vi "cRIO_FPGA_COMMUNICATION  Schreibe Werte für eine Station.vi"(8 "Fehler (Eingang, kein Fehler)":errorcluster, 9 "Stationen":bool[][](array[boolean]), 10 "Bänder":bool[][](array[boolean]), 11 "FPGA-VI-Referenz (Ausgang)":refnum<k20>) -> (0 "Fehler (Ausgang)":errorcluster)   [LabVIEW 2013, in "cRIO_FPGA_COMMUNICATION.lvlib"]
uses:
  cRIO_FPGA_COMMUNICATION.lvlib
  <vilib>/Utility/error.llb/Error Cluster From Error Code.vi
  <vilib>/rvi/errors/niLvFpgaAdjustHostInterfaceError.vi
  <vilib>/rvi/interface/nirviReadWriteControl/nirviReadWriteControl.xnode
  FPGA Bitfiles/Test_FPGATarget_CScRIOPBFPGADP-M_4E0AD52E.lvbitx
  NiFpgaLv.dll
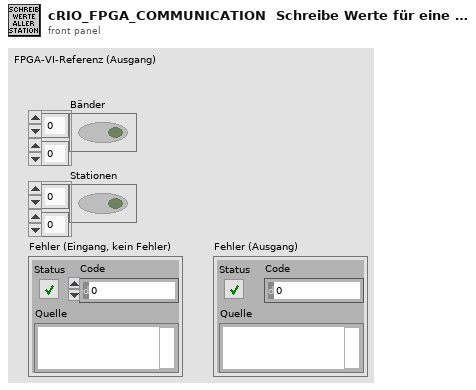
[diagram p1: front panel]
types:
  T1 = enum16{"Init", "Zählerkonfig. setzen", "lese Zählerkonfig."}
  T2 = enum16{"Init", "Zählerwert nullen", "Zählerwert setzen", "lese gesetzten Zählerwert"}
  T3 = cluster{"Index (Station/Band)":u8, "Station/Band":enum16{"Station", "Band"}, "Bitstelle":u8, "Zählrichtung":enum16{"Hochzählen", "Runterzählen"}}[]
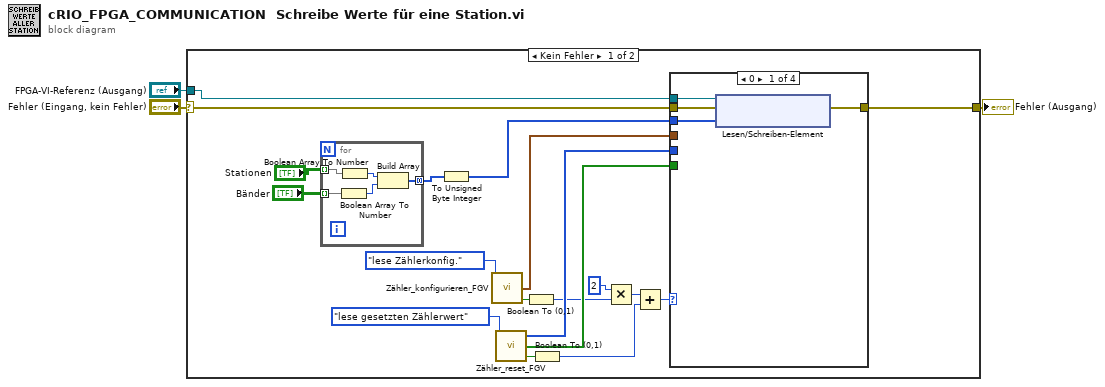
[diagram p0: block diagram]
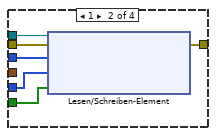
[diagram p2: hidden frame]
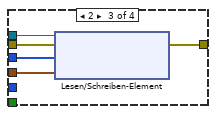
[diagram p3: hidden frame]
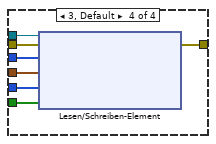
[diagram p4: hidden frame]
diagram:
  n1 = case shown="Kein Fehler" "Fehler (Eingang, kein Fehler)" {
    selector: "Fehler (Eingang, kein Fehler)" -> [w17 w50]
    tunnel: [w18 w50] -> w3
    tunnel: "FPGA-VI-Referenz (Ausgang)" -> [w16 _]
    frame No Error {
      n2 = for {
        tunnel: "Bänder" -> [w49] mode=indexing
        tunnel: "Stationen" -> [w48] mode=indexing
        tunnel: [w45] -> w20 mode=concatenating
        n3 = Boolean Array To Number(Boolean array=w49) -> (number=w47:u32)
        n4 = Boolean Array To Number(Boolean array=w48) -> (number=w46:u32)
        n5 = Build Array(w46, w47) -> (w45:u32[])
      }
      n6 = To Unsigned Byte Integer(number=w20) -> (unsigned 8bit integer=w19:u8[])
      n7 = call "Zähler_konfigurieren_FGV.vi"("Modus"=T1."lese Zählerkonfig.") -> ("Zählerkonfig."=w15:T3, "Werte verändert"=w9:bool)  [unwired: 5 in]
      n8 = call "Zähler_reset_FGV.vi"("Modus"=T2."lese gesetzten Zählerwert") -> ("Zählerwerte"=w13:u16[], "zurücksetzen"=w12:bool[], "Werte verändert"=w10:bool)  [unwired: 4 in]
      n9 = Boolean To (0,1)(Boolean=w9) -> (0, 1=w8:i16)
      n10 = Boolean To (0,1)(Boolean=w10) -> (0, 1=w6:i16)
      n11 = Multiply(x=i16 2, y=w8) -> (x*y=w5:i16)
      n12 = Add(x=w5, y=w6) -> (x+y=w4:i16)
      n13 = case shown="0" w4 {
        tunnel: w19 -> [w26 w32 w37 w44]
        tunnel: [w25 w31 w36 w43] -> w18
        tunnel: w17 -> [w24 w30 w35 w42]
        tunnel: w16 -> [w23 w29 w34 w41]
        tunnel: w15 -> [_ _ w33 w40]
        tunnel: w13 -> [_ w28 _ w39]
        tunnel: w12 -> [_ w27 _ w38]
        frame 0 {
          n14 = xnode "Lesen/Schreiben-Element"("FPGA-VI-Referenz (Eingang)"=w23, "Fehler (Eingang)"=w24, "Write output data:"=w26) -> ("Fehler (Ausgang)"=w25:errorcluster)  [unwired: 1 out]
        }
        frame 1 {
          n15 = xnode "Lesen/Schreiben-Element"("FPGA-VI-Referenz (Eingang)"=w29, "Fehler (Eingang)"=w30, "Write output data:"=w32, "zu setzender Zählerwert"=w28, "Zähler zurücksetzen"=w27) -> ("Fehler (Ausgang)"=w31:errorcluster)  [unwired: 1 out]
        }
        frame 2 {
          n16 = xnode "Lesen/Schreiben-Element"("FPGA-VI-Referenz (Eingang)"=w34, "Fehler (Eingang)"=w35, "Write output data:"=w37, "Zähler-Einstellung"=w33) -> ("Fehler (Ausgang)"=w36:errorcluster)  [unwired: 1 out]
        }
        frame 3, Default {
          n17 = xnode "Lesen/Schreiben-Element"("FPGA-VI-Referenz (Eingang)"=w41, "Fehler (Eingang)"=w42, "Write output data:"=w44, "Zähler-Einstellung"=w40, "zu setzender Zählerwert"=w39, "Zähler zurücksetzen"=w38) -> ("Fehler (Ausgang)"=w43:errorcluster)  [unwired: 1 out]
        }
      }
    }
    frame Error {
    }
  }
  "Fehler (Ausgang)" <- w3
